vi "Protected Read (0D U8).vi"(8 "error in (no error)":errorcluster, 9 "offset (0)":u64 format="%d bytes", 10 "value in":u8, 11 "Pointer in":refnum<class "Pointer.lvclass">) -> (0 "error out":errorcluster, 1 "offset out":u64 format="%d bytes", 2 "value out":u8, 3 "Pointer out":refnum<class "Pointer.lvclass">)   [LabVIEW 2016, in "Memory Manager.lvlib" / "Pointer.lvclass"]
doc: "Reads the contents of the address specified by <b>pointer + offset</b> into <b>value</b>.\n\n<b>Note:</b> This VI is <b>safe</b>.\n\nSafe means that this function evaluates the size parameter of <b>pointer</b> to ensure that is inbounds of allocated memory before peforming a memory read/write. Reading/writing more data to a pointer than it has allocated can corrupt or crash LabVIEW."
uses:
  Pointer.lvclass
  Read (0D U8).vi
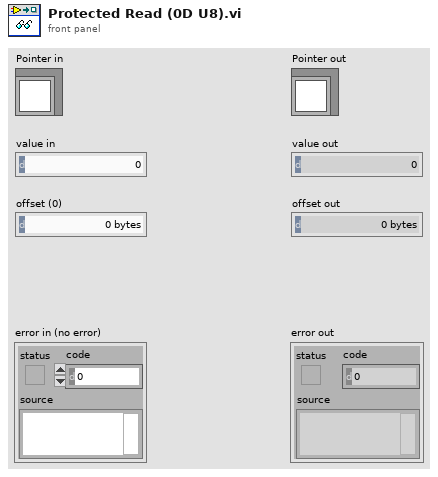
[diagram p1: front panel]
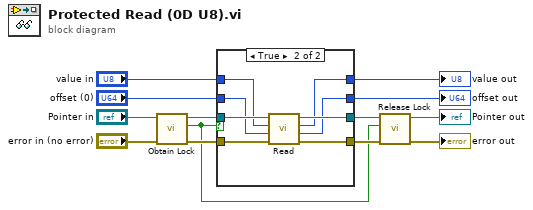
[diagram p0: block diagram]
diagram:
  n1 = call-dynamic "Obtain Lock.vi"("error in (no error)"="error in (no error)", "Pointer in"="Pointer in") -> ("error out"=w7:errorcluster, "lock status"=w1:bool, "Pointer out"=w8:refnum<class "Pointer.lvclass">)  [unwired: 6 in, 1 out]
  n2 = case shown="True" w1 {
    tunnel: [w17 w25] -> w13
    tunnel: [w14 w24] -> w12
    tunnel: [w15 w23] -> w11
    tunnel: w8 -> [w17 w22]
    tunnel: w7 -> [w16 w21]
    tunnel: "value in" -> [w14 w20]
    tunnel: "offset (0)" -> [w15 w19]
    tunnel: [w16 w18] -> w4
    frame False {
    }
    frame True {
      n3 = call-poly "Read.vi"("error in (no error)"=w21, "offset (0)"=w19, "value in"=w20, "Pointer in"=w22) -> ("error out"=w18:errorcluster, "offset out"=w23:u64, "value out"=w24:u8, "Pointer out"=w25:refnum<class "Pointer.lvclass">)  [unwired: 4 in]
    }
  }
  "value out" <- w12
  "offset out" <- w11
  n4 = call-dynamic "Release Lock.vi"("error in (no error)"=w4, "new lock status (T)"=w1, "Pointer in"=w13) -> ("error out"=→"error out":errorcluster, "Pointer out"=→"Pointer out":refnum<class "Pointer.lvclass">)  [unwired: 6 in, 1 out]
